vi "Process SwitchActionList.vi"(8 "error in (no error)":errorcluster, 10 "SwitchActionList":T1 {"RelayAction" items=["CloseRelay"=21, "OpenRelay"=20]}, 11 "Switch Action Processor In":refnum<class "Switch Action Processor.lvclass">) -> (0 "error out":errorcluster, 3 "Switch Action Processor Out":refnum<class "Switch Action Processor.lvclass">)   [LabVIEW 2015, in "SLSC Switch.lvlib" / "Switch Action Processor.lvclass"]
uses:
  Switch Action Processor.lvclass
  Unique String Buffer/Unique String Buffer.lvclass
  Relay/Relay.lvclass
  slscsl/RelayAction.ctl
  slscsl/slscsl.lvclass
  <vilib>/SLSC/SLSC.lvlib
  <vilib>/SLSC/Flatten Names (String).vi
  <vilib>/National Instruments/SLSC Local or Remote Interface/SLSC Interface Class/SLSC Interface.lvclass
  <vilib>/National Instruments/SLSC Local or Remote Interface/SLSC Interface Class/Set Generic Property/Set Generic Property (Bool).vi
  slscsl/SwitchAction.ctl
  slscsl/SwitchActionsArray.ctl
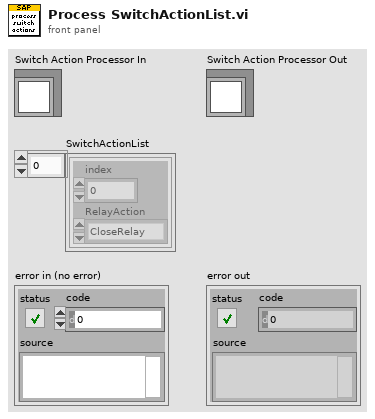
[diagram p1: front panel]
types:
  T1 = typedef "SLSC Switch.lvlib/slscsl.lvclass/SwitchActionsArray.ctl" = T2[]
  T2 = typedef "SLSC Switch.lvlib/slscsl.lvclass/SwitchAction.ctl" = cluster{"index":i32, "RelayAction":T3}
  T3 = typedef "SLSC Switch.lvlib/slscsl.lvclass/RelayAction.ctl" = u32
  T4 = typedef "SLSC Switch.lvlib/Relay.lvclass/Command.ctl" = cluster{"resource name":string, "command":refnum<k21>}
  T5 = typedef "SLSC Switch.lvlib/Relay.lvclass/Property.ctl" = cluster{"resource name":string, "property":refnum<k21>}
  T6 = typedef "SLSC Switch.lvlib/slscsl.lvclass/RelayPosition.ctl" = i32
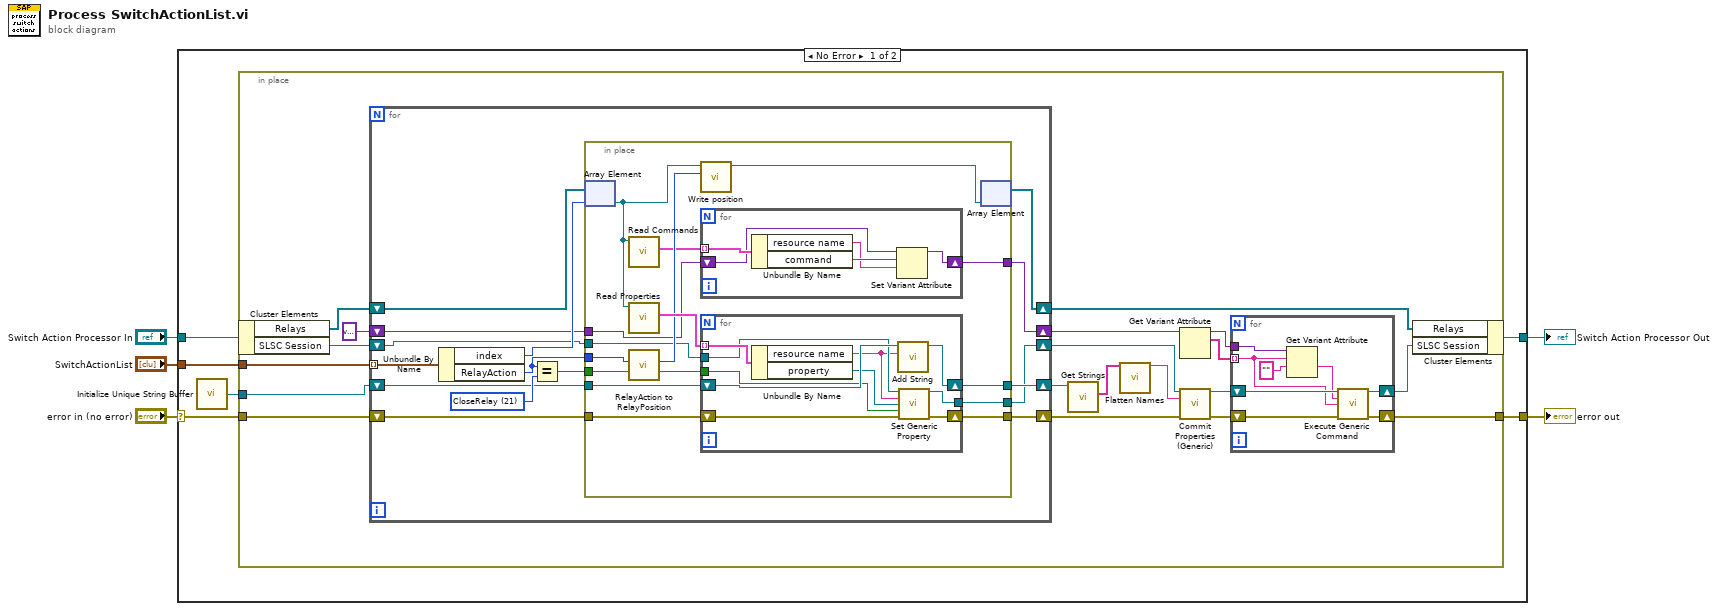
[diagram p0: block diagram]
diagram:
  n1 = case shown="No Error" "error in (no error)" {
    selector: "error in (no error)" -> [w9 w84]
    tunnel: "Switch Action Processor In" -> [w11 w85]
    tunnel: "SwitchActionList" -> [w10 _]
    tunnel: [w8 w85] -> w2
    tunnel: [w6 w84] -> w1
    frame No Error {
      n2 = call "Initialize Unique String Buffer.vi"() -> ("Buffer out"=w7:refnum<class "Unique String Buffer.lvclass">)  [unwired: 2 in]
      n3 = in-place {
        in-place-border: w10 -> [w30]
        in-place-border: w9 -> [w28]
        in-place-border: w7 -> [w26]
        in-place-border: [w12] -> w6
        n4 = in-place-cluster #1(w11) -> ("Relays"=w29:refnum<class "Relay.lvclass">[], "SLSC Session"=w19:refnum<class "SLSC Interface.lvclass">)
        n5 = for {
          tunnel: w30 -> [w53] mode=indexing
          shift-right: [w50] -> w27
          shift-left: w29 -> [w51]
          shift-right: [w45] -> w16
          shift-left: w28 -> [w47]
          shift-right: [w43] -> w25
          shift-left: w26 -> [w44]
          shift-right: [w41] -> w22
          shift-left: variant -> [w42]
          shift-right: [w39] -> w18
          shift-left: w19 -> [w40]
          w49 = T3 21 items=["CloseRelay"=21, "OpenRelay"=20] ("y")
          n6 = Unbundle By Name(w53) -> ("index"=w52:i32, "RelayAction"=w46:T3)
          n7 = Equal?(x=w46, y=w49) -> (x = y?=w48:bool)
          n8 = in-place {
            in-place-border: w48 -> [w67]
            in-place-border: w47 -> [w66]
            in-place-border: w46 -> [w63]
            in-place-border: [w62] -> w45
            in-place-border: w44 -> [w61]
            in-place-border: [w60] -> w43
            in-place-border: w42 -> [w57]
            in-place-border: [w56] -> w41
            in-place-border: w40 -> [w55]
            in-place-border: [w54] -> w39
            n9 = in-place-array #2(w51, w52) -> (w59:refnum<class "Relay.lvclass">)
            n10 = call "Read Commands.vi"("Relay in"=w59) -> ("Commands"=w58:T4[])  [unwired: 8 in, 2 out]
            n11 = call "Read Properties.vi"("Relay in"=w59) -> ("Properties"=w68:T5[])  [unwired: 8 in, 2 out]
            n12 = call "RelayAction to RelayPosition.vi"("action"=w63) -> ("position"=w64:T6)  [unwired: 10 in]
            n13 = call "Write position.vi"("position"=w64, "Relay in"=w59) -> ("Relay out"=w65:refnum<class "Relay.lvclass">)  [unwired: 8 in, 1 out]
            n14 = for {
              tunnel: w58 -> [w73] mode=indexing
              shift-right: [w69] -> w56
              shift-left: w57 -> [w70]
              n15 = Unbundle By Name(w73) -> ("resource name"=w71:string, "command"=w72:refnum<k21>)
              n16 = Set Variant Attribute(Variant=w70, name=w72, value=w71) -> (Variant out=w69:variant)  [unwired: 1 in, 2 out]
            }
            n17 = for {
              tunnel: w68 -> [w83] mode=indexing
              tunnel: w67 -> [w79]
              shift-right: [w76] -> w62
              shift-left: w66 -> [w78]
              shift-right: [w81] -> w60
              shift-left: w61 -> [w82]
              tunnel: w55 -> [w75]
              tunnel: [w77] -> w54
              n18 = Unbundle By Name(w83) -> ("resource name"=w74:string, "property"=w80:refnum<k21>)
              n19 = call "Add String.vi"("string"=w74, "Buffer in"=w82) -> ("Buffer out"=w81:refnum<class "Unique String Buffer.lvclass">)  [unwired: 8 in, 1 out]
              n20 = call-poly <vilib>:"Set Generic Property.vi"("SLSC Interface in"=w75, "devices"=w74, "property"=w80, "property value"=w79, "error in (no error)"=w78) -> ("SLSC Interface out"=w77:refnum<class "SLSC Interface.lvclass">, "error out"=w76:errorcluster)  [unwired: 9 in]
            }
            n21 = in-place-array #2(w65) -> (w50:refnum<class "Relay.lvclass">[])  [unwired: 1 out]
          }
        }
        n22 = call "Get Strings.vi"("Buffer in"=w25) -> ("strings"=w24:string[])  [unwired: 8 in, 2 out]
        n23 = call-poly <vilib>:"Flatten Names.vi"("names in"=w24) -> ("names out"=w17:string)  [unwired: 13 in, 1 out]
        n24 = Get Variant Attribute(Variant=w22) -> (duplicate Variant=w21:variant, names=w20:string[])  [unwired: 3 in, 2 out]
        n25 = call-dynamic "Commit Properties (Generic).vi"("SLSC Interface in"=w18, "resources"=w17, "error in (no error)"=w16) -> ("SLSC Interface out"=w15:refnum<class "SLSC Interface.lvclass">, "error out"=w13:errorcluster)  [unwired: 11 in]
        n26 = for {
          tunnel: w21 -> [w38]
          tunnel: w20 -> [w32] mode=indexing
          shift-right: [w33] -> w12
          shift-left: w13 -> [w34]
          shift-right: [w35] -> w14
          shift-left: w15 -> [w36]
          n27 = Get Variant Attribute(Variant=w38, name=w32, default value (empty Variant)="" ("resource name")) -> (value=w31:string)  [unwired: 1 in, 3 out]
          n28 = call-dynamic "Execute Generic Command.vi"("SLSC Interface in"=w36, "resources"=w31, "command"=w32, "error in (no error)"=w34) -> ("SLSC Interface out"=w35:refnum<class "SLSC Interface.lvclass">, "error out"=w33:errorcluster)  [unwired: 10 in]
        }
        n29 = in-place-cluster #1("Relays"=w27, "SLSC Session"=w14) -> (w8:refnum<class "Switch Action Processor.lvclass">)
      }
    }
    frame Error {
    }
  }
  "error out" <- w1
  "Switch Action Processor Out" <- w2
